vi "heds_custom_set_calibration.vi"() -> ()   [LabVIEW 2025]
uses:
  <userlib>/HOLOEYE SLM Display SDK 4.1.0/types/heds_slm_id_typedef.ctl
panel:
  out "error code 2":i32
  in  "vlow":dbl
  out "SLM ID out 2":T1
  out "error out 2":errorcluster
  out "error code":i32
  in  "vhigh":dbl
  in  "error in (no error)":errorcluster
  in  "SLM ID":T1
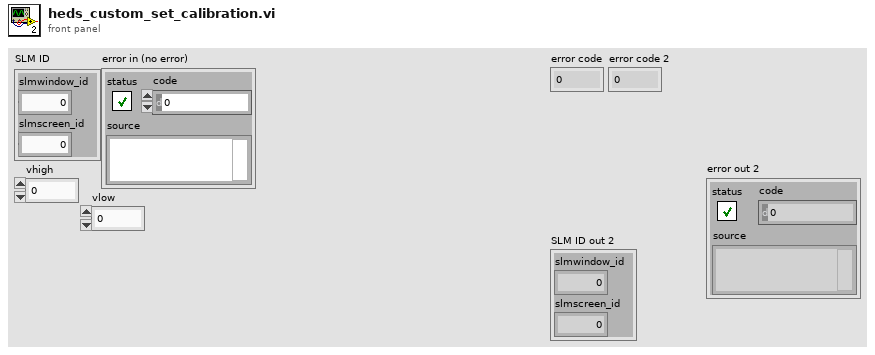
[diagram p1: front panel]
types:
  T1 = typedef "heds_slm_id_typedef.ctl" = cluster{"slmwindow_id":u32, "slmscreen_id":u32}
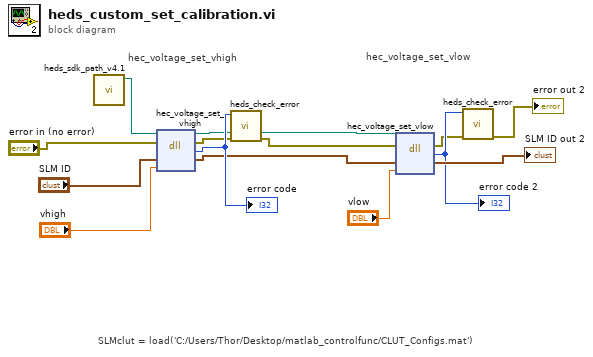
[diagram p0: block diagram]
diagram:
  # "SLMclut = load('C:/Users/Thor/Desktop/matlab_controlfunc/CLUT_Configs.mat')"
  # "hec_voltage_set_vlow"
  # "hec_voltage_set_vhigh"
  n1 = call <userlib>:"heds_sdk_path_v4.1.vi"() -> ("HEDS_LABVIEW_DLL_PATH"=w14:path)  [unwired: 9 in, 2 out]
  n2 = dll-call lib="holoeye_slmdisplaysdk.*" fn="hec_voltage_set_vhigh"(path in=w14, error in="error in (no error)", "slm_id"="SLM ID", "vhigh"="vhigh") -> (path out=w6:path, error out=w9:errorcluster, "error code"=w10:i32, "slm_id"=w8:T1)  [unwired: 2 in]
  "error code" <- w10
  n3 = call <userlib>:"heds_check_error.vi"("error in (no error)"=w9, "error code"=w10) -> ("error out"=w5:errorcluster)  [unwired: 8 in, 1 out]
  n4 = dll-call lib="holoeye_slmdisplaysdk.*" fn="hec_voltage_set_vlow"(path in=w6, error in=w5, "slm_id"=w8, "vlow"="vlow") -> (error out=w2:errorcluster, "error code"=w3:i32, "slm_id"=→"SLM ID out 2":T1)  [unwired: 2 in, 1 out]
  "error code 2" <- w3
  n5 = call <userlib>:"heds_check_error.vi"("error in (no error)"=w2, "error code"=w3) -> ("error out"=→"error out 2":errorcluster)  [unwired: 8 in, 1 out]
